vi "Configure Digital Signal Interface Module.vi"(6 "Loop Back Test (3: Device)":u16(ring)=3 items=["Digital Bus", "Cable", "N5102A", "Device"], 7 "Enable Digital Signal Interface Module (F:Disable)":bool, 8 "error in (no error)":errorcluster, 9 "Data Transmission Type (0: Parallel)":u16(ring) items=["Parallel", "Serial", "Parallel interleaving I/Q", "Parallel interleaving I", "Parallel interleaving Q/I"], 10 "Logic Data Type (5: 3.3 volt CMOS signal)":u16(ring)=5 items=["Low voltage differential signal", "Low voltage TTL signal", "1.5 volt CMOS signal", "1.8 volt CMOS signal", "2.5 volt CMOS signal", "3.3 volt CMOS signal", "Simple Serial Interface"], 11 "VISA resource name":refnum<visa-resource-name>) -> (0 "error out":errorcluster, 3 "VISA resource name out":refnum<visa-resource-name>)   [LabVIEW 2018, in "Agilent PSG MXG Series.lvlib"]
doc: "Configures digital signal interface module N5102A.\n\n<B>Notes:</B>\n(1) This VI is valid in E8267D that installs <B>Option 601</B> or <B>Option 602</B> (Internal baseband generator), and <B>Option 003</B> (PSG digital output connectivity with N5102A) or <B>Option 004</B> (PSG digital input connectivity with N5102A).\n(2) This VI is valid in N5172B/82B that with <B> Option 003</B> or <B>Option 004</B> or <B>both</B>."
uses:
  Agilent PSG MXG Series.lvlib
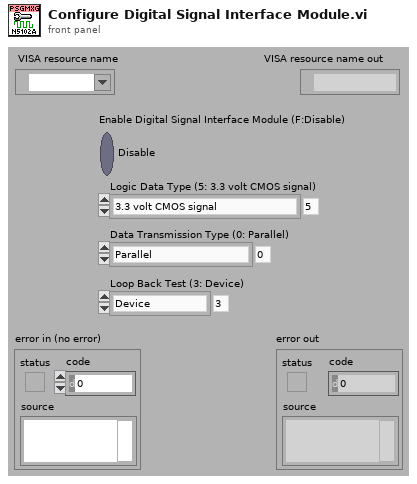
[diagram p1: front panel]
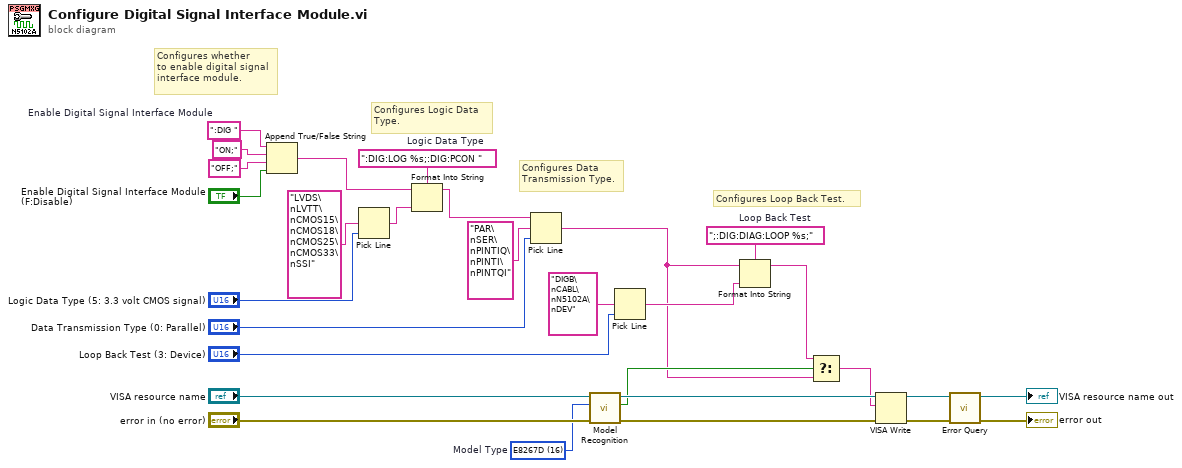
[diagram p0: block diagram]
diagram:
  w5 = u16 16 items=["N5181A"=0, "N5182A"=1, "N5183A"=2, "N5161A"=3, "N5162A"=4, "E8241A"=5, "E8244A"=6, "E8251A"=7, "E8254A"=8, "E8247C"=10, "E8257C"=11, "E8267C"=12, "E8257D"=15, "E8267D"=16, "N5171B"=17, "N5172B"=18, "N5181B"=19, "N5182B"=20, "N5173B"=21, "N5183B"=22]  # Model Type
  w17 = ";:DIG:DIAG:LOOP %s;"  # Loop Back Test
  w23 = ":DIG:LOG %s;:DIG:PCON "  # Logic Data Type
  w29 = ":DIG "  # Enable Digital Signal Interface Module
  # "Configures Loop Back Test."
  # "Configures Data\nTransmission Type."
  # "Configures Logic Data\nType."
  # "Configures whether\nto enable digital signal\ninterface module."
  n1 = Append True/False String(1:"Enable Digital Signal Interface Module (F:Disable)", 2:"OFF;" ("false string"), 3:"ON;" ("true string"), 4:w29) -> (0:w24:string)
  n2 = Pick Line(multi-line string="LVDS\nLVTT\nCMOS15\nCMOS18\nCMOS25\nCMOS33\nSSI", line index="Logic Data Type (5: 3.3 volt CMOS signal)") -> (output string=w22:string)  [unwired: 1 out]
  n3 = Format Into String(format string=w23, initial string=w24, w22) -> (resulting string=w20:string)  [unwired: 1 in, 1 out]
  n4 = Pick Line(string ("")=w20, multi-line string="PAR\nSER\nPINTIQ\nPINTI\nPINTQI", line index="Data Transmission Type (0: Parallel)") -> (output string=w2:string)
  n5 = call "Model Recognition.vi"("error in (no error)"="error in (no error)", "Model Type (0: N5181A)"=w5, "VISA resource name"="VISA resource name") -> ("error out"=w6:errorcluster, "Is Model Correct"=w4:bool, "VISA resource name out"=w7:refnum<visa-resource-name>)  [unwired: 6 out]
  n6 = Pick Line(multi-line string="DIGB\nCABL\nN5102A\nDEV", line index="Loop Back Test (3: Device)") -> (output string=w15:string)  [unwired: 1 out]
  n7 = Format Into String(format string=w17, initial string=w2, w15) -> (resulting string=w3:string)  [unwired: 1 in, 1 out]
  n8 = Select(t=w3, s=w4, f=w2) -> (s? t:f=w1:string)
  n9 = VISA Write(VISA resource name=w7, write buffer=w1, error in (no error)=w6) -> (VISA resource name out=w13:refnum<visa-resource-name>, error out=w12:errorcluster)  [unwired: 1 out]
  n10 = call "Error Query.vi"("error in (no error)"=w12, "VISA resource name"=w13) -> ("error out"=→"error out":errorcluster, "VISA resource name out"=→"VISA resource name out":refnum<visa-resource-name>)  [unwired: 8 out]
